vi "cm_Check SW Overload.vi"(0 "Display State In":T3={"Chan"=[], "First Drop?"=TRUE, "Notifier Name"="", "Refresh View"=FALSE, "Scale to Input Range"=FALSE, "Linear View"=FALSE, "Display"={"Current"=6618880, "Peak"=6618880}, "Property/Method"=enum."No Update", "Time Display Ref"=[]}, 5 "Overload Threshold":dbl=90.0, 9 "Container State":T5, 11 "error in (no error)":errorcluster) -> (4 "Display State Out":T3={"Chan"=[], "First Drop?"=TRUE, "Notifier Name"="", "Refresh View"=FALSE, "Scale to Input Range"=FALSE, "Linear View"=FALSE, "Display"={"Current"=6618880, "Peak"=6618880}, "Property/Method"=enum."No Update", "Time Display Ref"=[]}, 6 "Overloaded Channels":T2(array[cluster]), 8 "Overload Detected":bool, 15 "error out":errorcluster)   [LabVIEW 2009, in "Channel Monitor [System].xctl"]
doc: "Check for any channels whose peak has been above some threshold. The threshold is set in % of input range for the channel. This is purely a software overload detection and does not perform hardware overload detection."
uses:
  Channel Monitor [System].xctl
  <vilib>/_xctls/Container State.ctl
  subVIs/cm_Channel Monitor State.ctl
  TypeDef/cm_Property_Method.ctl
  <vilib>/_xctls/XControlSupport.lvlib
panel:
  in  "Overloaded Channels 2":T1
  in  "Overloaded Channels":T2(array[cluster])
  # "Add Controls & Indicators that form the parameters of the method here. Hook them to the connector pane. Do not delete the controls & indicators that are already hooked to the connector pane.\n \nTo setup the parameters  for this method, right click on this item in the Project Tree & select \"Configure Method...\"."
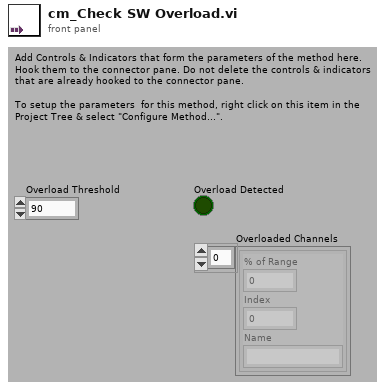
[diagram p1: front panel]
types:
  T1 = cluster{"% of Range":dbl, "Index":i32, "Name":string}
  T2 = cluster{"% of Range":dbl, "Index":i32, "Name":string}[]
  T3 = typedef "Channel Monitor [System].xctl/cm_Channel Monitor State.ctl" = cluster{"Chan":cluster{"ChanName":string, "Current":dbl, "Peak":dbl, "Input Range":dbl}[], "First Drop?":bool, "Notifier Name":string, "Refresh View":bool, "Scale to Input Range":bool, "Linear View":bool, "Display":cluster{"Current":u32, "Peak":u32}, "Property/Method":T4, "Time Display Ref":refnum<vi>[]}
  T4 = typedef "Channel Monitor [System].xctl/cm_Property_Method.ctl" = enum16{"No Update", "Color: Currrent", "Color: Peak", "Close Time Displays"}
  T5 = typedef "XControlSupport.lvlib/Container State.ctl" = cluster{"Indicator?":bool, "Run Mode?":bool, " Refnum":refnum<vi>}
  T6 = cluster{"ChanName":string, "Current":dbl, "Peak":dbl, "Input Range":dbl}[]
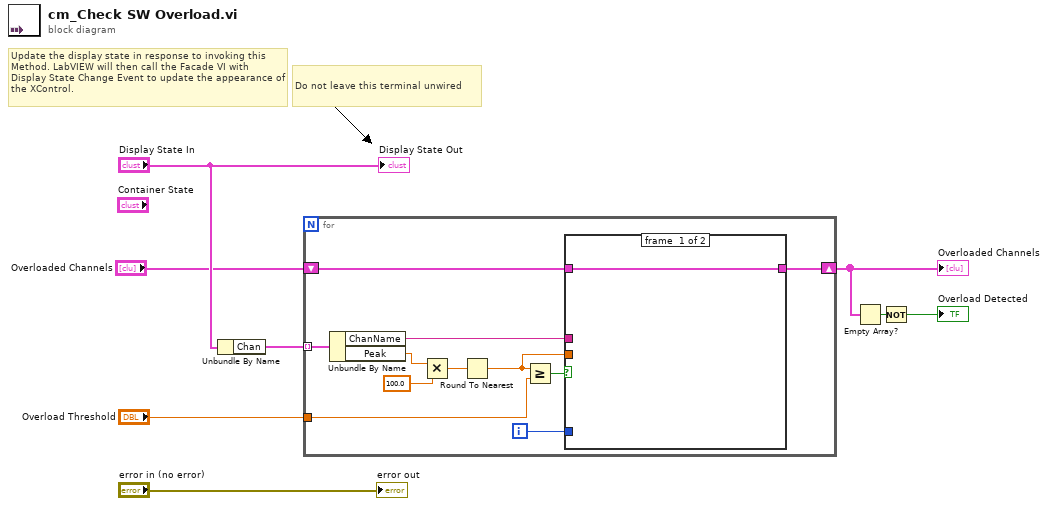
[diagram p0: block diagram]
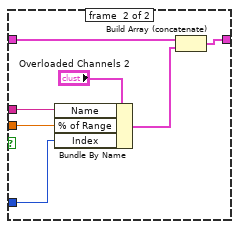
[diagram p2: hidden frame]
diagram:
  # "Do not leave this terminal unwired"
  # "Update the display state in response to invoking this Method. LabVIEW will then call the Facade VI with Display State Change Event to update the appearance of the XControl."
  n1 = Unbundle By Name("Display State In") -> ("Chan"=w6:T6)
  n2 = for {
    tunnel: w6 -> [w11] mode=indexing
    shift-right: [w13] -> w1
    shift-left: "Overloaded Channels" -> [w14]
    tunnel: "Overload Threshold" -> [w18]
    i -> [w15]
    n3 = Unbundle By Name(w11) -> ("ChanName"=w16:string, "Peak"=w12:dbl)
    n4 = Multiply(x=w12, y=100.0) -> (x*y=w10:dbl)
    n5 = Round To Nearest(number=w10) -> (nearest integer value=w9:dbl)
    n6 = Greater Or Equal?(x=w9, y=w18) -> (x >= y?=w17:bool)
    n7 = case shown="True" w17 {
      tunnel: w9 -> [_ w27]
      tunnel: w16 -> [_ w26]
      tunnel: w15 -> [_ w25]
      tunnel: w14 -> [w20 w24]
      tunnel: [w20 w23] -> w13
      frame #0 {
      }
      frame #1 {
        n8 = Bundle By Name(cluster="Overloaded Channels 2", "Name"=w26, "% of Range"=w27, "Index"=w25) -> (w22:T1)
        n9 = Build Array (concatenate)(w24, w22) -> (w23:T2)
      }
    }
  }
  "Overloaded Channels" <- w1
  n10 = Empty Array?(array=w1) -> (empty?=w3:bool)
  n11 = Not(x=w3) -> (.not. x?=→"Overload Detected":bool)
  "Display State Out" <- "Display State In"
  "error out" <- "error in (no error)"
